vi "Configure Trigger (Width).vi"(0 "VISA resource name":refnum<visa-resource-name>, 1 "Polarity (0:Positive)":u16(ring) items=["Positive", "Negative"], 2 "Upper Limit (5E-6s)":dbl=5e-06, 3 "Lower Limit (2E-6s)":dbl=2e-06, 5 "Source (0:Channel1)":u16(ring) items=["Channel1", "Channel2", "Channel3", "Channel4", "Digital Channel0", "Digital Channel1", "Digital Channel2", "Digital Channel3", "Digital Channel4", "Digital Channel5", "Digital Channel6", "Digital Channel7", "Digital Channel8", "Digital Channel9", "Digital Channel10", "Digital Channel11", "Digital Channel12", "Digital Channel13", "Digital Channel14", "Digital Channel15"], 7 "Trigger Level(0V)":dbl, 9 "Trigger Condition (0:Inside)":u16(ring) items=["Inside", "Outside"], 11 "error in (no error)":errorcluster, 12 "Trigger If Width (0:Occurs)":u16(ring) items=["Occurs", "Logic"], 13 "Trigger Event (0:A Event)":u16(ring) items=["A Event", "B Event"]) -> (4 "VISA resource name out":refnum<visa-resource-name>, 6 "Trigger Event Out":u16(ring) items=["A Event", "B Event"], 15 "error out":errorcluster)   [LabVIEW 2015, in "Tektronix 7000 Series.lvlib"]
doc: "Configures width trigger settings for an oscilloscope. A width trigger occurs when the oscilloscope detects a positive or negative pulse with a width between or outside the thresholds you specify.\n\n<B>Note:</B> \nTDS5000 ,TDS5000B,TDS6000 ,CSA7000 and TDS7000 series oscilloscopes don't support B Width Trigger."
uses:
  <instrlib>/Tektronix 7000 Series/Tektronix 7000 Series.lvlib
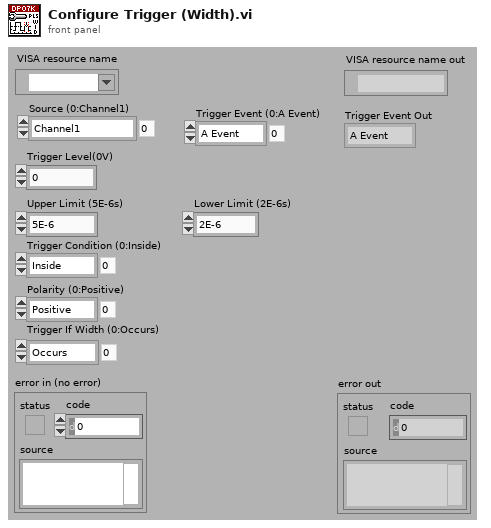
[diagram p1: front panel]
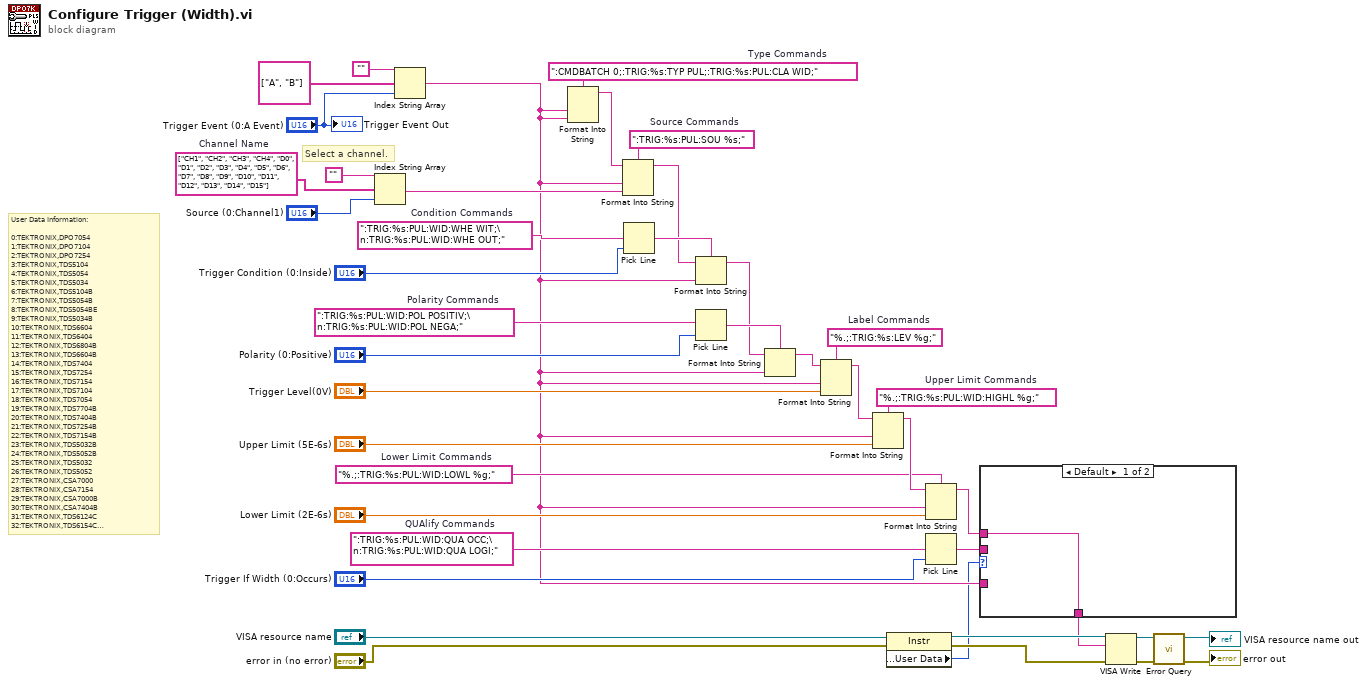
[diagram p0: block diagram]
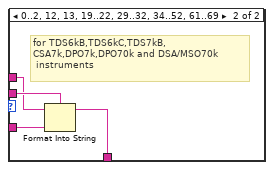
[diagram p2: hidden frame]
diagram:
  w2 = string[] ["CH1", "CH2", "CH3", "CH4", "D0", "D1", "D2", "D3", "D4", "D5", "D6", "D7", "D8", "D9", "D10", "D11", "D12", "D13", "D14", "D15"]  # Channel Name
  w23 = "%.;:TRIG:%s:PUL:WID:LOWL %g;"  # Lower Limit Commands
  w26 = ":TRIG:%s:PUL:WID:QUA OCC;\n:TRIG:%s:PUL:WID:QUA LOGI;"  # QUAlify Commands
  w27 = ":TRIG:%s:PUL:WID:POL POSITIV;\n:TRIG:%s:PUL:WID:POL NEGA;"  # Polarity Commands
  w29 = ":TRIG:%s:PUL:WID:WHE WIT;\n:TRIG:%s:PUL:WID:WHE OUT;"  # Condition Commands
  w28 = "%.;:TRIG:%s:PUL:WID:HIGHL %g;"  # Upper Limit Commands
  w30 = "%.;:TRIG:%s:LEV %g;"  # Label Commands
  w31 = ":TRIG:%s:PUL:SOU %s;"  # Source Commands
  w22 = ":CMDBATCH 0;:TRIG:%s:TYP PUL;:TRIG:%s:PUL:CLA WID;"  # Type Commands
  # "User Data Information:\n\n0:TEKTRONIX,DPO7054\n1:TEKTRONIX,DPO7104\n2:TEKTRONIX,DPO7254\n3:TEKTRONIX,TDS5104\n4:TEKTRONIX,TDS5054\n5:TEKTRONIX,TDS5034\n6:TEKTRONIX,TDS5104B\n7:TEKTRONIX,TDS5054B\n8:TEKTRONIX,TDS5054BE\n9:TEKTRONIX,TDS5034B\n10:TEKTRONIX,TDS6604\n11:TEKTRONIX,TDS6404\n12:TEKTRONIX,TDS6804B\n13:TEKTRONIX,TDS6604B\n14:TEKTRONIX,TDS7404\n15:TEKTRONIX,TDS7254\n16:TEKTRONIX,TDS7154\n17:TEKTRONIX,TDS7104\n18:TEKTRONIX,TDS7054\n19:TEKTRONIX,TDS7704B\n20:TEKTRONIX,TDS7404B\n21:TEKTRONIX,TDS7254B\n22:TEKTRONIX,TDS7154B\n23:TEKTRONIX,TDS5032B\n24:TEKTRONIX,TDS5052B\n25:TEKTRONIX,TDS5032\n26:TEKTRONIX,TDS5052\n27:TEKTRONIX,CSA7000\n28:TEKTRONIX,CSA7154\n29:TEKTRONIX,CSA7000B\n30:TEKTRONIX,CSA7404B\n31:TEKTRONIX,TDS6124C\n32:TEKTRONIX,TDS6154C\n33:TEKTRONIX,CSA7404\n34:TEKTRONIX,DPO70404\n35:TEKTRONIX,DPO70604\n36:TEKTRONIX,DPO70804\n37:TEKTRONIX,DSA70404\n38:TEKTRONIX,DSA70604\n39:TEKTRONIX,DSA70804\n40:TEKTRONIX,DPO7354\n41:TEKTRONIX,DPO71254\n42:TEKTRONIX,DPO71604\n43:TEKTRONIX,DPO72004\n44:TEKTRONIX,DSA71254\n45:TEKTRONIX,DSA71604\n46:TEKTRONIX,DSA72004\n47:TEKTRONIX,MSO70404\n48:TEKTRONIX,MSO70604\n49:TEKTRONIX,MSO70804\n50:TEKTRONIX,MSO71254\n51:TEKTRONIX,MSO71604\n52:TEKTRONIX,MSO72004\n53:TEKTRONIX,MSO5034\n54:TEKTRONIX,MSO5054\n55:TEKTRONIX,MSO5104\n56:TEKTRONIX,MSO5204\n57:TEKTRONIX,DPO5034\n58:TEKTRONIX,DPO5054\n59:TEKTRONIX,DPO5104\n60:TEKTRONIX,DPO5204\n61: TEKTRONIX,DPO71254C\n62: TEKTRONIX,DPO71604C\n63: TEKTRONIX,DPO72004C\n64: TEKTRONIX,DSA71254C\n65: TEKTRONIX,DSA71604C\n66: TEKTRONIX,DSA72004C\n67: TEKTRONIX,MSO71254C\n68: TEKTRONIX,MSO71604C\n69: TEKTRONIX,MSO72004C"
  # "Select a channel."
  n1 = Index String Array(1:"Source (0:Channel1)", 2:w2, 3:"") -> (0:w21:string)
  n2 = Index String Array(1:"Trigger Event (0:A Event)", 2:string[] ["A", "B"], 3:"" ("Empty String Constant")) -> (0:w10:string)
  n3 = Format Into String(format string=w22, w10, w10) -> (resulting string=w20:string)  [unwired: 2 in, 1 out]
  n4 = Format Into String(format string=w31, initial string=w20, w10, w21) -> (resulting string=w18:string)  [unwired: 1 in, 1 out]
  n5 = Pick Line(multi-line string=w29, line index="Trigger Condition (0:Inside)") -> (output string=w19:string)  [unwired: 1 in]
  n6 = Format Into String(format string=w19, initial string=w18, w10) -> (resulting string=w16:string)  [unwired: 1 in, 1 out]
  n7 = Pick Line(multi-line string=w27, line index="Polarity (0:Positive)") -> (output string=w17:string)  [unwired: 1 in]
  n8 = Format Into String(format string=w17, initial string=w16, w10) -> (resulting string=w11:string)  [unwired: 1 in, 1 out]
  n9 = Format Into String(format string=w30, initial string=w11, w10, "Trigger Level(0V)") -> (resulting string=w25:string)  [unwired: 1 in, 1 out]
  n10 = Format Into String(format string=w28, initial string=w25, w10, "Upper Limit (5E-6s)") -> (resulting string=w24:string)  [unwired: 1 in, 1 out]
  n11 = property class="Instr"(reference="VISA resource name", error in="error in (no error)") -> (reference out=w7:refnum<visa-resource-name>, error out=w6:errorcluster, "General Settings:User Data"=w5:u32)
  n12 = Format Into String(format string=w23, initial string=w24, w10, "Lower Limit (2E-6s)") -> (resulting string=w4:string)  [unwired: 1 in, 1 out]
  n13 = Pick Line(multi-line string=w26, line index="Trigger If Width (0:Occurs)") -> (output string=w15:string)  [unwired: 1 in]
  n14 = case shown="Default" w5 {
    tunnel: w15 -> [_ w47]
    tunnel: w10 -> [_ w46]
    tunnel: w4 -> [w43 w45]
    tunnel: [w43 w44] -> w3
    frame Default {
    }
    frame 0..2, 12, 13, 19..22, 29..32, 34..52, 61..69 {
      # "for TDS6kB,TDS6kC,TDS7kB,\nCSA7k,DPO7k,DPO70k and DSA/MSO70k\n instruments"
      n15 = Format Into String(format string=w47, initial string=w45, w46) -> (resulting string=w44:string)  [unwired: 1 in, 1 out]
    }
  }
  n16 = VISA Write(VISA resource name=w7, write buffer=w3, error in (no error)=w6) -> (VISA resource name out=w38:refnum<visa-resource-name>, error out=w37:errorcluster)  [unwired: 1 out]
  n17 = call <instrlib>:"Error Query.vi"("error in (no error)"=w37, "VISA resource name"=w38) -> ("error out"=→"error out":errorcluster, "VISA resource name out"=→"VISA resource name out":refnum<visa-resource-name>)  [unwired: 6 in, 2 out]
  "Trigger Event Out" <- "Trigger Event (0:A Event)"
